vi "General setup bundler-String.vi"(7 "Section":string, 8 "error in (no error)":errorcluster, 10 "String":T2, 11 "Setup.ini ref":T1) -> (0 "error out":errorcluster, 3 "Setup.ini ref":T1)   [LabVIEW 2013]
uses:
  <vilib>/Utility/config.llb/Config Data RefNum.ctl
  Typedefs/Ini file interface (String).ctl
  <vilib>/Utility/config.llb/NI_LVConfig.lvlib
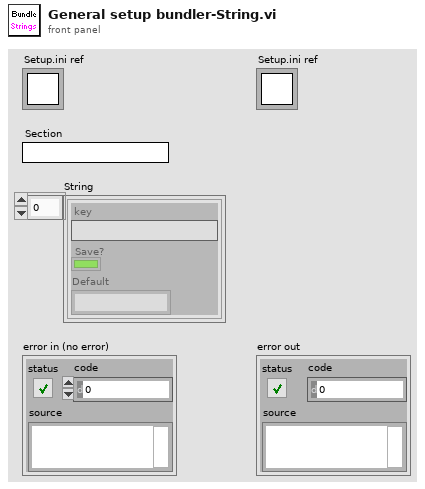
[diagram p1: front panel]
types:
  T1 = typedef "NI_LVConfig.lvlib/Config Data RefNum.ctl" = refnum<k1>
  T2 = typedef "Ini file interface (String).ctl" = cluster{"key":string, "Save?":bool, "Default":string}[]
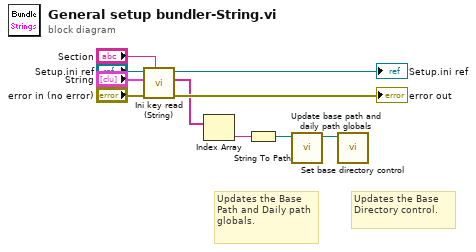
[diagram p0: block diagram]
diagram:
  # "Updates the Base Path and Daily path globals."
  # "Updates the Base Directory control."
  n1 = call "Ini key read (String).vi"("Section name"="Section", "error in (no error)"="error in (no error)", "Keys setup"="String", "Ini file ref in"="Setup.ini ref") -> ("error out"=→"error out":errorcluster, "Value read/used"=w7:string[], "Ini file ref"=→"Setup.ini ref":T1)  [unwired: 5 in]
  n2 = Index Array(array=w7) -> (element=w3:string)  [unwired: 1 in]
  n3 = String To Path(string=w3) -> (path=w2:path)
  n4 = call "Update base path and daily path globals.vi"("Base Directory"=w2) -> ("Base Directory (dupl)"=w1:path)  [unwired: 9 in, 1 out]
  n5 = call "Set base directory control.vi"("Base path"=w1) -> ()  [unwired: 10 in, 1 out]
